vi "1 Tap 48-Bit RGB.vi"() -> (0 "Pixels":cluster{"Pixel 0":u64})   [LabVIEW 2013]
uses:
  <vilib>/rvi/eio/common/nirviEmuTemplateMethod_errors.vi
  <vilib>/eio/EIONode/EIONode.xnode
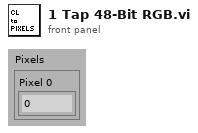
[diagram p1: front panel]
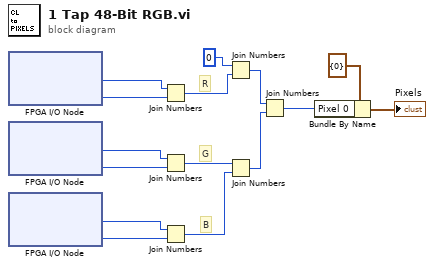
[diagram p0: block diagram]
diagram:
  # "B"
  # "R"
  # "G"
  n1 = xnode "FPGA I/O Node"() -> ("CL Port B"=w6:u8, "CL Port A"=w15:u8)  [unwired: 2 in, 2 out]
  n2 = xnode "FPGA I/O Node"() -> ("CL Port E"=w5:u8, "CL Port D"=w9:u8)  [unwired: 2 in, 2 out]
  n3 = xnode "FPGA I/O Node"() -> ("CL Port F"=w4:u8, "CL Port C"=w8:u8)  [unwired: 2 in, 2 out]
  n4 = Join Numbers(hi=w6, lo=w15) -> ((hi.lo)=w14:u16)
  n5 = Join Numbers(hi=w5, lo=w9) -> ((hi.lo)=w13:u16)
  n6 = Join Numbers(hi=w4, lo=w8) -> ((hi.lo)=w7:u16)
  n7 = Join Numbers(hi=u16 0, lo=w14) -> ((hi.lo)=w11:u32)
  n8 = Join Numbers(hi=w13, lo=w7) -> ((hi.lo)=w10:u32)
  n9 = Join Numbers(hi=w11, lo=w10) -> ((hi.lo)=w2:u64)
  n10 = Bundle By Name(cluster=cluster{"Pixel 0":u64} {"Pixel 0"=0} ("Data"), "Pixel 0"=w2) -> (→"Pixels":cluster{"Pixel 0":u64})
